vi "Read Topic Registry.vi"(8 "error in":errorcluster, 11 "Broker in":refnum<class "Broker.lvclass">) -> (0 "error out":errorcluster, 2 "Topic Registry":T1[](array[typedef]), 3 "Broker out":refnum<class "Broker.lvclass">)   [LabVIEW 2014, in "Broker.lvclass"]
uses:
  Broker.lvclass
  Controls/Topic Ref.ctl
  Broker.lvclass/Broker.ctl
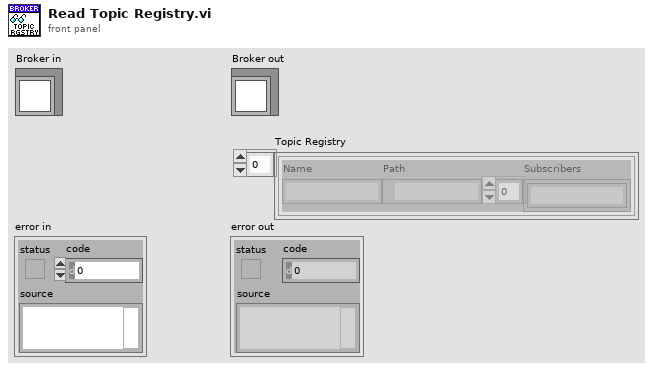
[diagram p1: front panel]
types:
  T1 = typedef "Topic Ref.ctl" = cluster{"Name":string, "Path":path, "Subscribers":string[]}
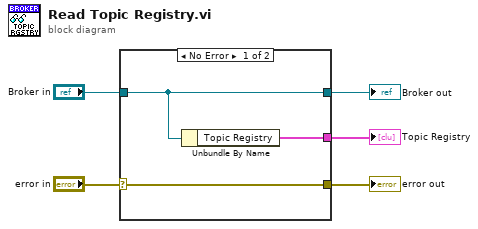
[diagram p0: block diagram]
diagram:
  n1 = case shown="No Error" "error in" {
    selector: "error in" -> [w8 w9]
    tunnel: [w8 w9] -> w4
    tunnel: [w7 w10] -> w2
    tunnel: "Broker in" -> [w7 w10]
    tunnel: [w6 _] -> w1
    frame No Error {
      n2 = Unbundle By Name(w7) -> ("Topic Registry"=w6:T1[])
    }
    frame Error {
    }
  }
  "error out" <- w4
  "Broker out" <- w2
  "Topic Registry" <- w1
